vi "LuaVIEW Flat Data.vi"() -> (0 "pass":bool)   [LabVIEW 2012]
uses:
  typedefs/t_LuaVIEW Reference.ctl
  subvis/private/LuaVIEW Pull (string).vi
  subvis/private/LuaVIEW Push (flat data).vi
  subvis/private/LuaVIEW Pull (boolean).vi
  subvis/private/LuaVIEW Pull (flat data).vi
  subvis/private/LuaVIEW Push (string).vi
  subvis/private/LuaVIEW Push (path).vi
  subvis/private/LuaVIEW Pull (path).vi
  subvis/private/LuaVIEW Pull (U32).vi
  subvis/private/LuaVIEW Push (refnum).vi
panel:
  in  "test path":path=path "c:/foo/bar/baz"
  in  "script file":path=path "scripts/flat data test.lua"
  out "hex type string on pulling":string
  out "pulled raw data string":string
  out "pull variant":variant
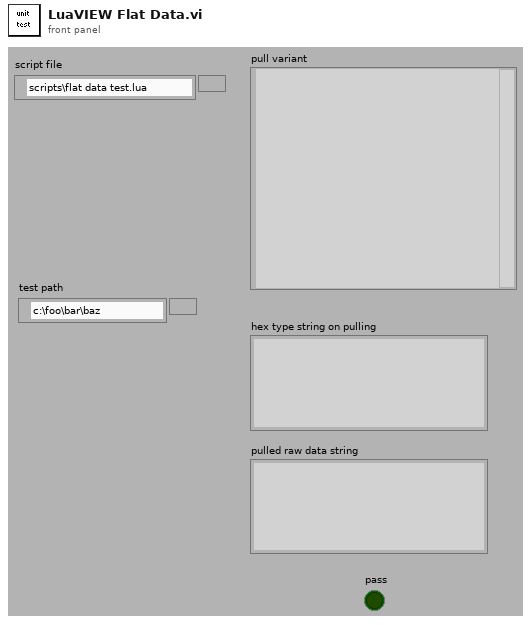
[diagram p1: front panel]
types:
  T1 = enum32{"execute", "initialize", "any:data=push(str:type,str:flat,[bool:order])", "str:flat=pull(str:type,any:data)", "str:flat=default(str:type,str:def,[any:data])", "str:item=pull_enum(str:item)", "push_pull_path()", "str:outpath=pull_push_path(str:inpath)", "ref:r=push_refnum(U32:num)", "print([any:thing],...)", "cleanup"}
  T2 = typedef "t_LuaVIEW Reference.ctl" = refnum<k1>
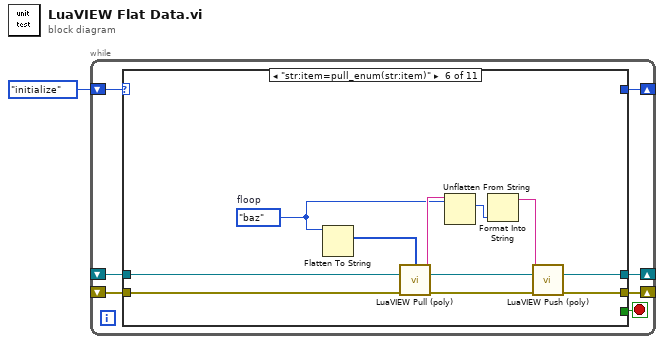
[diagram p0: block diagram]
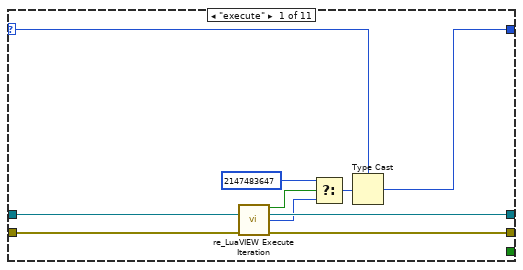
[diagram p2: hidden frame]
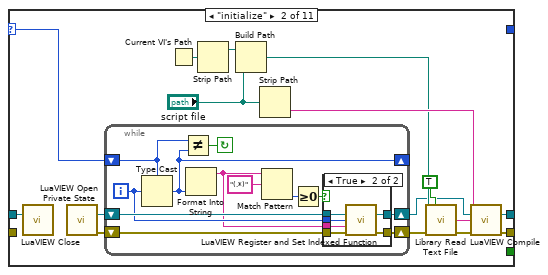
[diagram p3: hidden frame]
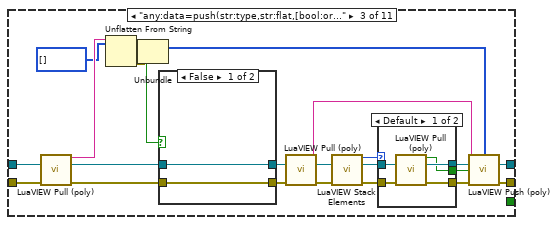
[diagram p5: hidden frame]
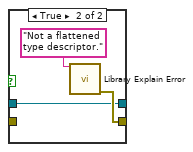
[diagram p7: hidden frame]
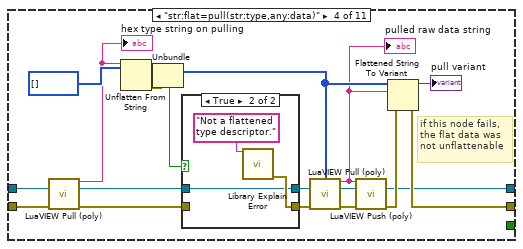
[diagram p8: hidden frame]
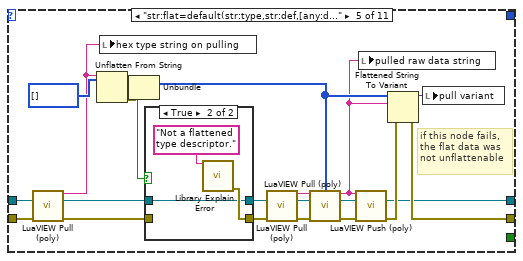
[diagram p10: hidden frame]
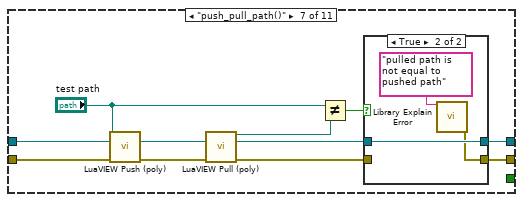
[diagram p12: hidden frame]
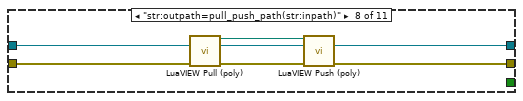
[diagram p14: hidden frame]
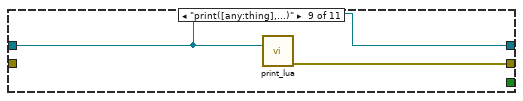
[diagram p15: hidden frame]
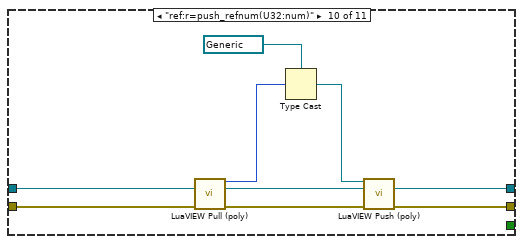
[diagram p16: hidden frame]
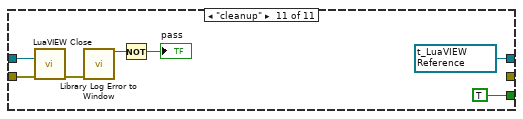
[diagram p17: hidden frame]
diagram:
  n1 = while {
    shift-right: [w6] -> _
    shift-left: T1."initialize" -> [w8]
    shift-right: [w4] -> _
    shift-left: _ -> [w5]
    shift-right: [w3] -> _
    shift-left: _ -> [w2]
    stop <- w7 stop-if-true
    n2 = case shown="\"str:item=pull_enum(str:item)\"" w8 {
      selector: w8 -> [w11 w30 _ _ _ _ _ _ _ _ _]
      tunnel: [_ _ _ _ _ _ _ _ _ _ TRUE] -> w7
      tunnel: [w9 _ _ _ _ _ _ _ _ _ _] -> w6
      tunnel: w5 -> [w18 w34 w75 w105 w131 w147 w154 w168 w172 w176 w189]
      tunnel: [w15 w31 w68 w93 w121 w143 w156 w165 w172 w174 w188] -> w4
      tunnel: [w16 w29 w67 w94 w122 w142 w157 w166 w173 w175 _] -> w3
      tunnel: w2 -> [w17 _ w76 w106 w132 w146 w153 w167 _ w177 w186]
      frame "execute" {
        n3 = call "re_LuaVIEW Execute Iteration.vi"("LuaVIEW reference in"=w18, "init or indexed function error"=w17) -> ("last?"=w13:bool, "LuaVIEW reference out"=w15:T2, "function index"=w14:i32, "final error"=w16:errorcluster)  [unwired: 10 in]
        n4 = Select(t=2147483647, s=w13, f=w14) -> (s? t:f=w10:i32)
        n5 = Type Cast(type=w11, x=w10) -> (*(type *) &x=w9:T1)
      }
      frame "initialize" {
        n6 = call "LuaVIEW Close.vi"("LuaVIEW reference"=w34) -> ()  [unwired: 14 in, 1 out]
        n7 = call "LuaVIEW Open Private State.vi"() -> ("LuaVIEW reference"=w32:T2, "error out"=w33:errorcluster)  [unwired: 14 in]
        n8 = while {
          shift-right: [w40] -> w24
          shift-left: w33 -> [w43]
          shift-right: [w41] -> w19
          shift-left: w32 -> [w42]
          shift-right: [w35] -> _
          shift-left: w30 -> [w36]
          i -> [w39]
          stop <- w46 continue-if-true
          n9 = Type Cast(type=w36, x=w39) -> (*(type *) &x=w35:T1)
          n10 = Not Equal?(x=w36, y=w35) -> (x != y?=w46:bool)
          n11 = Format Into String(w35) -> (resulting string=w37:string)  [unwired: 3 in, 1 out]
          n12 = Match Pattern(string=w37, regular expression="(.*)") -> (offset past match=w44:i32)  [unwired: 1 in, 3 out]
          n13 = Greater Or Equal To 0?(x=w44) -> (x >= 0?=w38:bool)
          n14 = case shown="True" w38 {
            tunnel: w42 -> [w48 w51]
            tunnel: w39 -> [_ w52]
            tunnel: w37 -> [_ w49]
            tunnel: [w47 w54] -> w40
            tunnel: [w48 w53] -> w41
            tunnel: w43 -> [w47 w50]
            frame False {
            }
            frame True {
              n15 = call "LuaVIEW Register and Set Indexed Function.vi"("LuaVIEW reference in"=w51, "index"=w52, "synopsis"=w49, "error in (no error)"=w50) -> ("LuaVIEW reference out"=w53:T2, "error out"=w54:errorcluster)  [unwired: 10 in]
            }
          }
        }
        n16 = Current VI's Path() -> (path=w28:path)
        n17 = Strip Path(path=w28) -> (stripped path=w27:path)  [unwired: 1 out]
        n18 = Build Path(base path=w27, name or relative path="script file") -> (appended path=w22:path)
        n19 = Strip Path(path="script file") -> (name=w25:string)  [unwired: 1 out]
        n20 = call "Library Read Text File.vi"("file path"=w22, "convert eol (F)"=TRUE, "error in (no error)"=w24) -> ("read text"=w20:string, "error out"=w23:errorcluster)  [unwired: 10 in, 1 out]
        n21 = call "LuaVIEW Compile.vi"("script name"=w25, "LuaVIEW reference in"=w19, "script"=w20, "error in (no error)"=w23) -> ("LuaVIEW reference out"=w31:T2, "error out"=w29:errorcluster)  [unwired: 10 in]
      }
      frame "any:data=push(str:type,str:flat,[bool:order])" {
        n22 = call-poly "LuaVIEW Pull (poly).vi"("LuaVIEW reference in"=w75, "error in (no error)"=w76) -> ("string"=w73:string, "LuaVIEW reference out"=w69:T2, "error out"=w70:errorcluster)  [unwired: 11 in]
        n23 = Unflatten From String(type=i16[] [] ("type descriptor"), binary string=w73) -> (value=w74:i16[], error out=w55:errorcluster)  [unwired: 3 in, 1 out]
        n24 = Unbundle(w55) -> ("status"=w71:bool)  [unwired: 2 out]
        n25 = case shown="False" w71 {
          tunnel: [w85 w88] -> w66
          tunnel: w70 -> [w85 _]
          tunnel: w69 -> [w84 w86]
          tunnel: [w84 w86] -> w65
          frame False {
          }
          frame True {
            n26 = call "Library Explain Error.vi"("explanation prefix (none)"="Not a flattened type descriptor.") -> ("explained error"=w88:errorcluster)  [unwired: 14 in]
          }
        }
        n27 = call-poly "LuaVIEW Pull (poly).vi"("LuaVIEW reference in"=w65, "error in (no error)"=w66) -> ("string"=w64:string, "LuaVIEW reference out"=w63:T2, "error out"=w62:errorcluster)  [unwired: 11 in]
        n28 = call "LuaVIEW Stack Elements.vi"("LuaVIEW reference in"=w63, "error in (no error)"=w62) -> ("elements"=w61:i32, "LuaVIEW reference out"=w57:T2, "error out"=w60:errorcluster)  [unwired: 11 in]
        n29 = case shown="Default" w61 {
          tunnel: w60 -> [w80 w83]
          tunnel: [w79 w83] -> w59
          tunnel: w57 -> [w81 w82]
          tunnel: [w78 w82] -> w58
          tunnel: [w77 _] -> w56
          frame Default {
            n30 = call-poly "LuaVIEW Pull (poly).vi"("LuaVIEW reference in"=w81, "error in (no error)"=w80) -> ("boolean"=w77:bool, "LuaVIEW reference out"=w78:T2, "error out"=w79:errorcluster)  [unwired: 11 in]
          }
          frame 0 {
          }
        }
        n31 = call-poly "LuaVIEW Push (poly).vi"("flat data"=w64, "type descriptor"=w74, "LuaVIEW reference in"=w58, "include cluster order (false)"=w56, "error in (no error)"=w59) -> ("LuaVIEW reference out"=w68:T2, "error out"=w67:errorcluster)  [unwired: 9 in]
      }
      frame "str:flat=pull(str:type,any:data)" {
        # "if this node fails,\nthe flat data was\nnot unflattenable"
        n32 = call-poly "LuaVIEW Pull (poly).vi"("LuaVIEW reference in"=w105, "error in (no error)"=w106) -> ("string"=w90:string, "LuaVIEW reference out"=w97:T2, "error out"=w99:errorcluster)  [unwired: 11 in]
        "hex type string on pulling" <- w90
        n33 = Unflatten From String(type=i16[] [] ("type descriptor"), binary string=w90) -> (value=w96:i16[], error out=w89:errorcluster)  [unwired: 3 in, 1 out]
        n34 = Unbundle(w89) -> ("status"=w101:bool)  [unwired: 2 out]
        n35 = case shown="True" w101 {
          tunnel: [w108 w111] -> w100
          tunnel: w99 -> [w108 _]
          tunnel: w97 -> [w107 w109]
          tunnel: [w107 w109] -> w98
          frame False {
          }
          frame True {
            n36 = call "Library Explain Error.vi"("explanation prefix (none)"="Not a flattened type descriptor.") -> ("explained error"=w111:errorcluster)  [unwired: 14 in]
          }
        }
        n37 = call-poly "LuaVIEW Pull (poly).vi"("type descriptor"=w96, "LuaVIEW reference in"=w98, "error in (no error)"=w100) -> ("flat data"=w91:string, "LuaVIEW reference out"=w102:T2, "error out"=w103:errorcluster)  [unwired: 10 in]
        "pulled raw data string" <- w91
        n38 = call-poly "LuaVIEW Push (poly).vi"("string"=w91, "LuaVIEW reference in"=w102, "error in (no error)"=w103) -> ("LuaVIEW reference out"=w93:T2, "error out"=w95:errorcluster)  [unwired: 11 in]
        n39 = Flattened String To Variant(4:w95, 6:w91, 7:w96) -> (0:w94:errorcluster, 3:→"pull variant":variant)
      }
      frame "str:flat=default(str:type,str:def,[any:data])" {
        # "if this node fails,\nthe flat data was\nnot unflattenable"
        n40 = call-poly "LuaVIEW Pull (poly).vi"("LuaVIEW reference in"=w131, "error in (no error)"=w132) -> ("string"=w118:string, "LuaVIEW reference out"=w125:T2, "error out"=w126:errorcluster)  [unwired: 11 in]
        n41 = Unflatten From String(type=i16[] [] ("type descriptor"), binary string=w118) -> (value=w124:i16[], error out=w112:errorcluster)  [unwired: 3 in, 1 out]
        n42 = local write "hex type string on pulling"(w118) -> ()
        n43 = Unbundle(w112) -> ("status"=w127:bool)  [unwired: 2 out]
        n44 = case shown="True" w127 {
          tunnel: [w134 w137] -> w114
          tunnel: w126 -> [w134 _]
          tunnel: w125 -> [w133 w135]
          tunnel: [w133 w135] -> w113
          frame False {
          }
          frame True {
            n45 = call "Library Explain Error.vi"("explanation prefix (none)"="Not a flattened type descriptor.") -> ("explained error"=w137:errorcluster)  [unwired: 14 in]
          }
        }
        n46 = call-poly "LuaVIEW Pull (poly).vi"("LuaVIEW reference in"=w113, "error in (no error)"=w114) -> ("string"=w117:string, "LuaVIEW reference out"=w116:T2, "error out"=w115:errorcluster)  [unwired: 11 in]
        n47 = call-poly "LuaVIEW Pull (poly).vi"("default flat data"=w117, "type descriptor"=w124, "LuaVIEW reference in"=w116, "error in (no error)"=w115) -> ("flat data"=w119:string, "LuaVIEW reference out"=w128:T2, "error out"=w129:errorcluster)  [unwired: 9 in]
        n48 = call-poly "LuaVIEW Push (poly).vi"("string"=w119, "LuaVIEW reference in"=w128, "error in (no error)"=w129) -> ("LuaVIEW reference out"=w121:T2, "error out"=w123:errorcluster)  [unwired: 11 in]
        n49 = local write "pulled raw data string"(w119) -> ()
        n50 = Flattened String To Variant(4:w123, 6:w119, 7:w124) -> (0:w122:errorcluster, 3:w120:variant)
        n51 = local write "pull variant"(w120) -> ()
      }
      frame "str:item=pull_enum(str:item)" {
        w138 = enum16{"foo", "bar", "baz"}."baz"  # floop
        n52 = Flatten To String(anything=w138) -> (type string=w148:i16[])  [unwired: 3 in, 2 out]
        n53 = call-poly "LuaVIEW Pull (poly).vi"("type descriptor"=w148, "LuaVIEW reference in"=w147, "error in (no error)"=w146) -> ("flat data"=w141:string, "LuaVIEW reference out"=w144:T2, "error out"=w145:errorcluster)  [unwired: 10 in]
        n54 = Unflatten From String(type=w138, binary string=w141) -> (value=w140:enum16{"foo", "bar", "baz"})  [unwired: 3 in, 2 out]
        n55 = Format Into String(w140) -> (resulting string=w139:string)  [unwired: 3 in, 1 out]
        n56 = call-poly "LuaVIEW Push (poly).vi"("string"=w139, "LuaVIEW reference in"=w144, "error in (no error)"=w145) -> ("LuaVIEW reference out"=w143:T2, "error out"=w142:errorcluster)  [unwired: 11 in]
      }
      frame "push_pull_path()" {
        n57 = call-poly "LuaVIEW Push (poly).vi"("path"="test path", "LuaVIEW reference in"=w154, "error in (no error)"=w153) -> ("LuaVIEW reference out"=w151:T2, "error out"=w152:errorcluster)  [unwired: 11 in]
        n58 = call-poly "LuaVIEW Pull (poly).vi"("LuaVIEW reference in"=w151, "error in (no error)"=w152) -> ("path"=w150:path, "LuaVIEW reference out"=w155:T2, "error out"=w158:errorcluster)  [unwired: 11 in]
        n59 = Not Equal?(x="test path", y=w150) -> (x != y?=w159:bool)
        n60 = case shown="True" w159 {
          tunnel: w158 -> [w160 _]
          tunnel: [w160 w163] -> w157
          tunnel: w155 -> [w161 w164]
          tunnel: [w161 w164] -> w156
          frame False {
          }
          frame True {
            n61 = call "Library Explain Error.vi"("explanation prefix (none)"="pulled path is not equal to pushed path") -> ("explained error"=w163:errorcluster)  [unwired: 14 in]
          }
        }
      }
      frame "str:outpath=pull_push_path(str:inpath)" {
        n62 = call-poly "LuaVIEW Pull (poly).vi"("LuaVIEW reference in"=w168, "error in (no error)"=w167) -> ("path"=w171:path, "LuaVIEW reference out"=w170:T2, "error out"=w169:errorcluster)  [unwired: 11 in]
        n63 = call-poly "LuaVIEW Push (poly).vi"("path"=w171, "LuaVIEW reference in"=w170, "error in (no error)"=w169) -> ("LuaVIEW reference out"=w165:T2, "error out"=w166:errorcluster)  [unwired: 11 in]
      }
      frame "print([any:thing],...)" {
        n64 = call "print_lua.vi"("LuaVIEW reference in"=w172) -> ("error out"=w173:errorcluster)  [unwired: 14 in]
      }
      frame "ref:r=push_refnum(U32:num)" {
        n65 = call-poly "LuaVIEW Pull (poly).vi"("LuaVIEW reference in"=w176, "error in (no error)"=w177) -> ("U32"=w179:u32, "LuaVIEW reference out"=w178:T2, "error out"=w180:errorcluster)  [unwired: 11 in]
        n66 = Type Cast(type=refnum<vi> refnum ("refnum"), x=w179) -> (*(type *) &x=w181:refnum<vi>)
        n67 = call-poly "LuaVIEW Push (poly).vi"("refnum"=w181, "LuaVIEW reference in"=w178, "error in (no error)"=w180) -> ("LuaVIEW reference out"=w174:T2, "error out"=w175:errorcluster)  [unwired: 11 in]
      }
      frame "cleanup" {
        w188 = T2 refnum items=["LuaVIEW"] ("LuaVIEW reference")
        n68 = call "LuaVIEW Close.vi"("LuaVIEW reference"=w189, "error in (no error)"=w186) -> ("dup error"=w185:errorcluster)  [unwired: 13 in]
        n69 = call "Library Log Error to Window.vi"("error in (no error)"=w185) -> ("error?"=w184:bool)  [unwired: 13 in, 1 out]
        n70 = Not(x=w184) -> (.not. x?=→"pass":bool)
      }
    }
  }
